vi "Re-tag Larvae v2 (SubVI).vi"(0 "Image Size":T2={"Height"=512, "Width"=512} {"Width" step=8; "Height" step=8}, 1 "BG SUB TH":i16=20, 2 "Subtract BG":bool, 3 "BG Image":u8[][](array[numeric]), 4 "vReset":refnum<queue>, 5 "Data In":T1, 6 "Range":cluster{"Lower value":u8, "Upper value":u8}={"Lower value"=100, "Upper value"=255}, 7 "flipFlag":refnum<queue>, 8 "Box Side":cluster{"Low":u32, "High":u32}={"Low"=16, "High"=96}, 10 "Box W + L":cluster{"Low":u32, "High":u32}={"Low"=40, "High"=150}, 12 "Area":cluster{"Low":u32, "High":u32}={"Low"=448, "High"=1280}) -> (14 "# of Objects":i32, 16 "BBOX Array":u64[](array[numeric]), 19 "HT LOC":u64[](array[numeric]))   [LabVIEW 2020]
uses:
  Controls (HOST)/Image Size.ctl
  Controls (HOST)/Data to Disk Bundle.ctl
  <vilib>/vision/NI_Vision_Development_Module.lvlib
panel:
  in  "Range":cluster{"Lower value":u8, "Upper value":u8}={"Lower value"=100, "Upper value"=255}
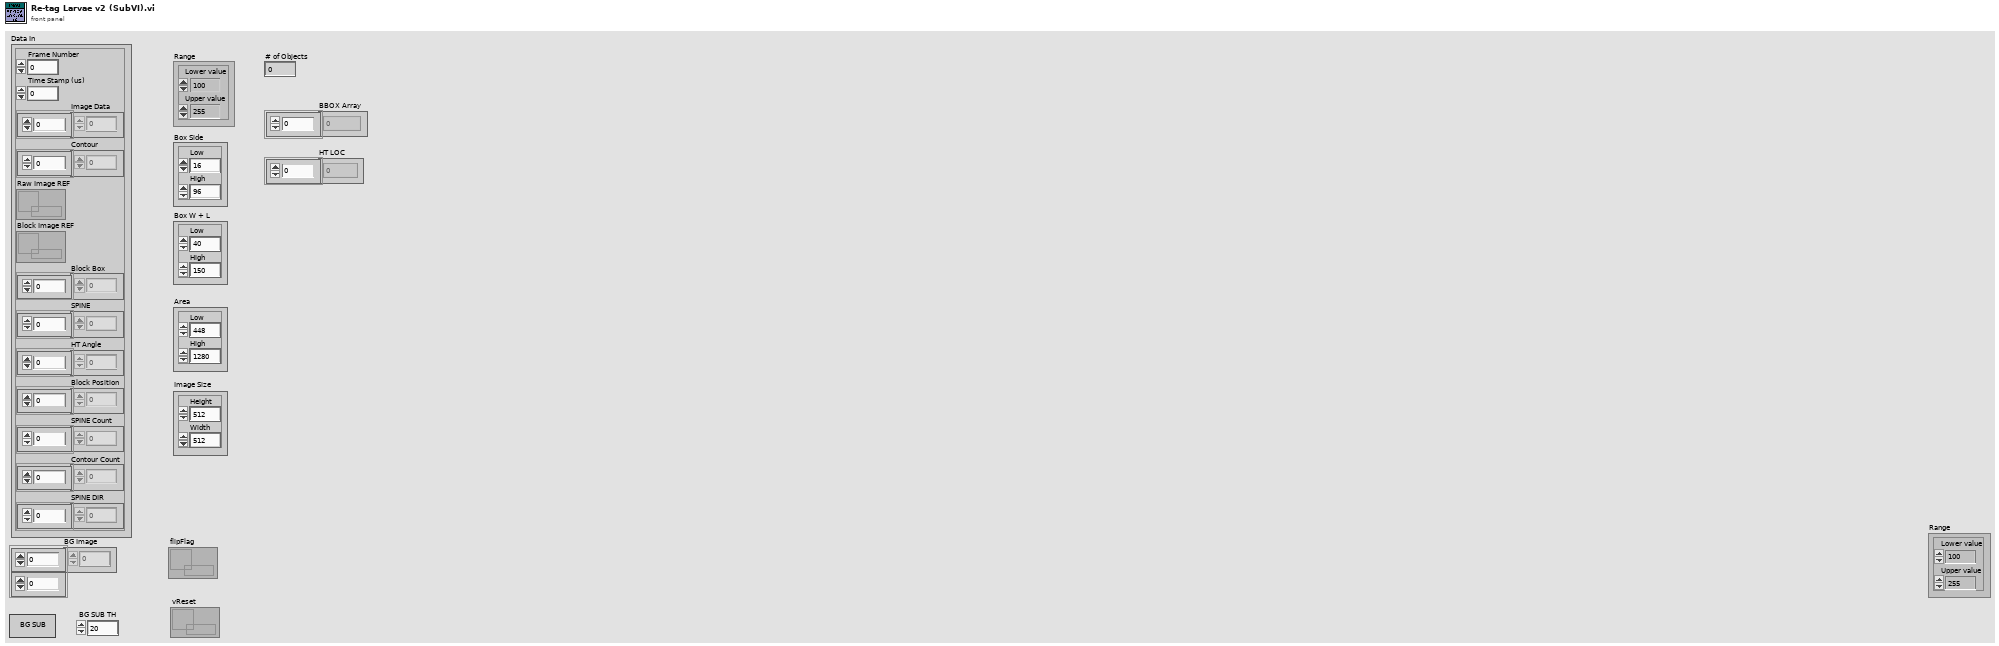
[diagram p1: front panel]
types:
  T1 = typedef "Data to Disk Bundle.ctl" = cluster{"Frame Number":u64, "Time Stamp (us)":u64, "Image Data":u64[], "Contour":u32[], "Raw Image REF":refnum<data-value>, "Block Image REF":refnum<data-value>, "Block Box":u64[], "SPINE":u32[], "HT Angle":u64[], "Block Position":u64[], "SPINE Count":u32[], "Contour Count":u32[], "SPINE DIR":u8[]}
  T2 = typedef "Image Size.ctl" = cluster{"Height":u16, "Width":u16}
  T3 = enum16{"big-endian, network order", "native, host order", "little-endian"}
  T4 = typedef "IMAQ Image.ctl" = refnum<image>
  T5 = cluster{"Area":dbl, "Number of Holes":dbl, "Bounding Rect":cluster{"Left":dbl, "Top":dbl, "Right":dbl, "Bottom":dbl}, "Center of Mass":cluster{"X":dbl, "Y":dbl}, "Orientation":dbl, "Dimensions":cluster{"Width":dbl, "Height":dbl}}[]
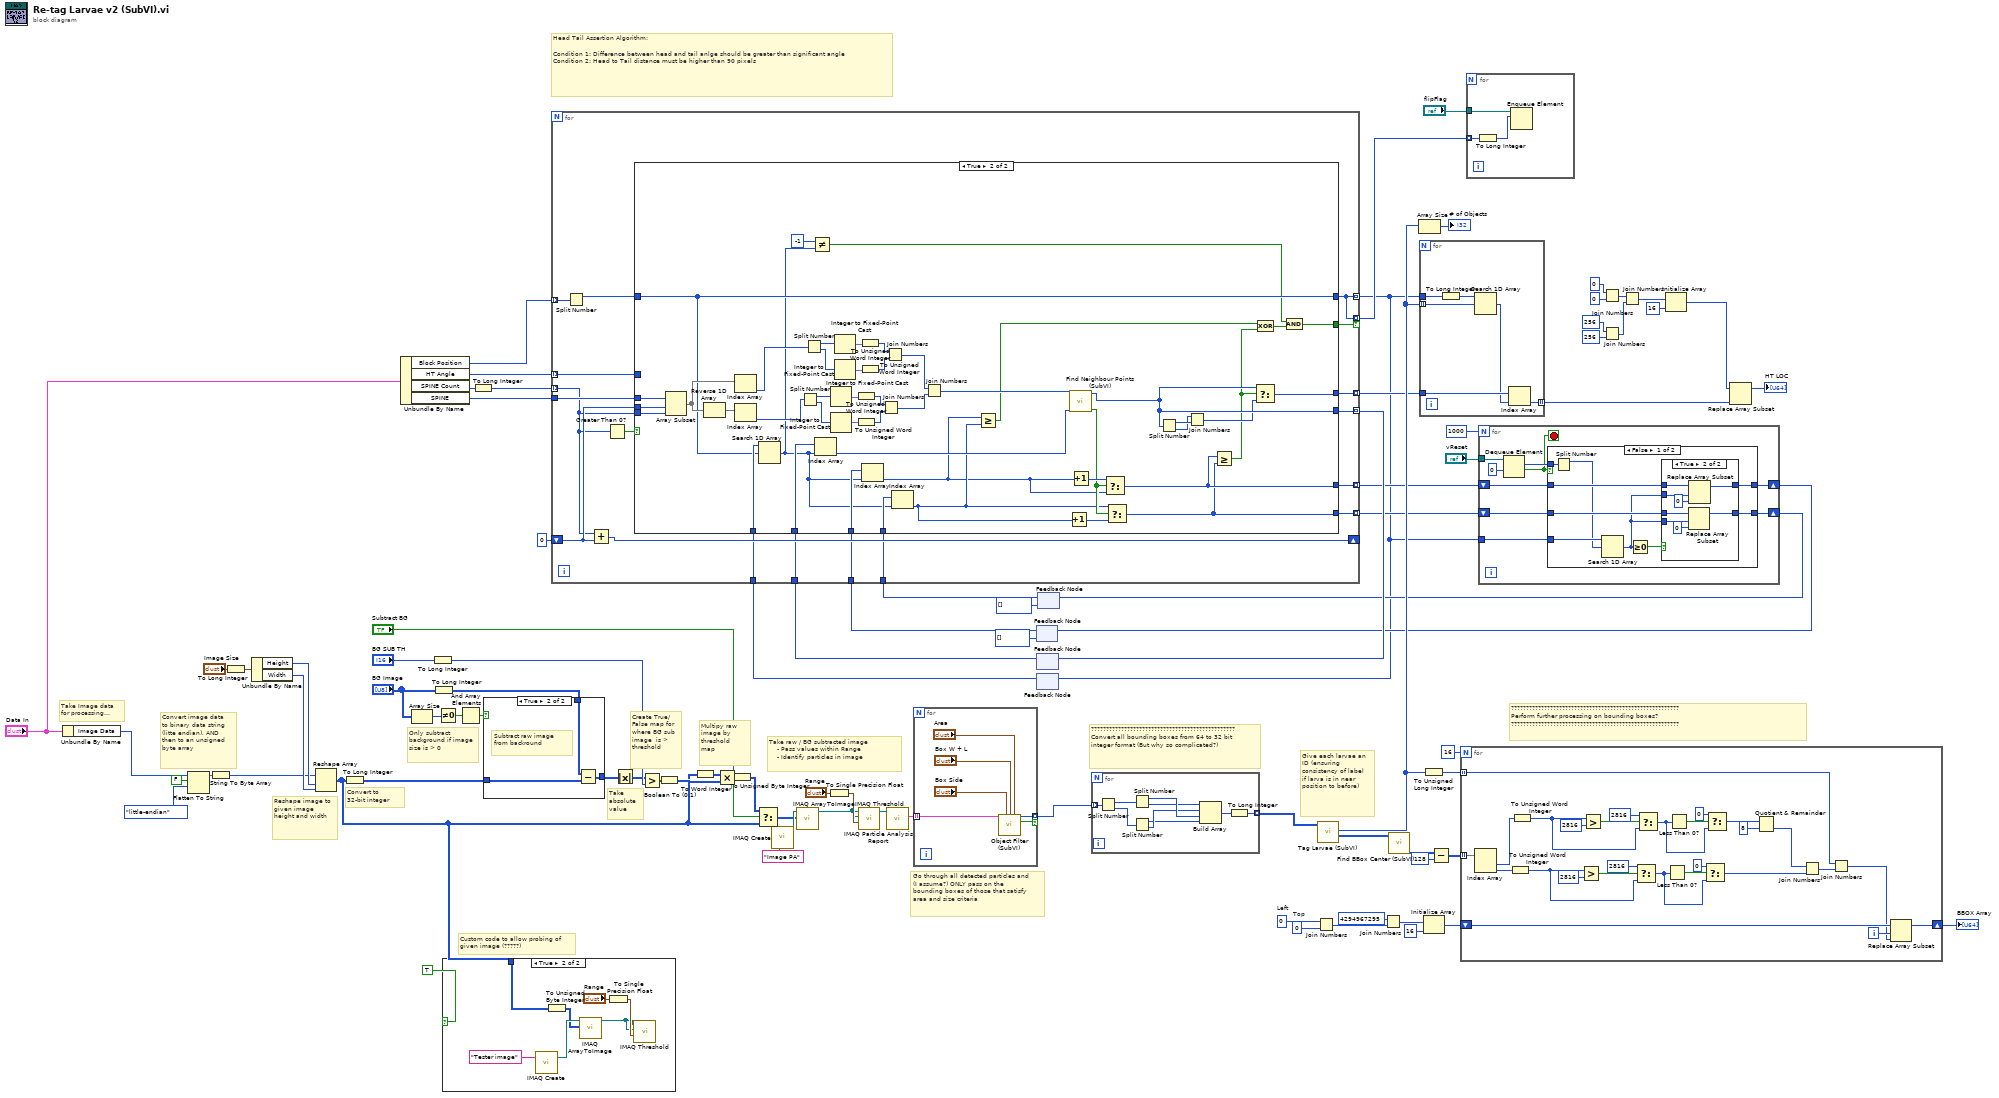
[diagram p0: block diagram]
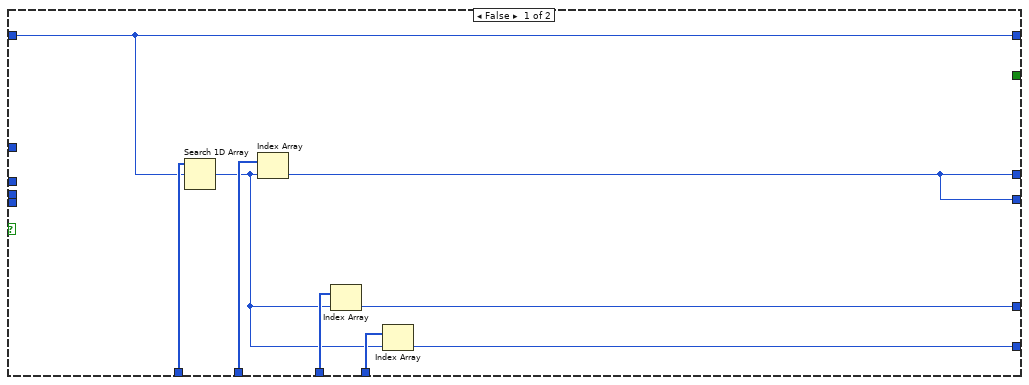
[diagram p5: hidden frame]
diagram:
  w71 = u16 0  # Left
  w67 = u16 0  # Top
  # "????????????????????????????????????????????????????????\nPerform further processing on bounding boxes?\n????????????????????????????????????????????????????????"
  # "Give each larvae an ID (ensuring consistency of label if larva is in near position to before)"
  # "????????????????????????????????????????????????\nConvert all bounding boxes from 64 to 32 bit integer format (But why so complicated?)"
  # "Go through all detected particles and (I assume?) ONLY pass on the bounding boxes of those that satisfy area and size criteria"
  # "Take raw / BG subtracted image\n    - Pass values within Range\n    - Identify particles in image"
  # "Multipy raw image by threshold map"
  # "Create True/False map for where BG sub image  is > threshold"
  # "Take absolute value"
  # "Custom code to allow probing of given image (?????)"
  # "Only subtract background if image size is > 0"
  # "Convert to 32-bit integer"
  # "Reshape image to given image height and width"
  # "Convert image data to binary data string (litte endian), AND then to an unsigned byte array"
  # "Take Image data for processing..."
  # "Head Tail Assertion Algorithm:\n\nCondition 1: Difference between head and tail anlge should be greater than significant angle\nCondition 2: Head to Tail distance must be higher than 90 pixels"
  n1 = Unbundle By Name("Data In") -> ("Image Data"=w58:u64[])
  n2 = Flatten To String(anything=w58, prepend array or string size? (T)=FALSE, byte order (0:big-endian, network order)=T3."little-endian") -> (data string=w55:string)  [unwired: 1 in, 2 out]
  n3 = String To Byte Array(string=w55) -> (unsigned byte array=w45:u8[])
  n4 = To Long Integer(number="Image Size") -> (32bit integer=w51:cluster{"Height":i32, "Width":i32})
  n5 = Unbundle By Name(w51) -> ("Height"=w53:i32, "Width"=w52:i32)
  n6 = Reshape Array(w45, w53, w52) -> (w1:u8[][])
  n7 = To Long Integer(number=w1) -> (32bit integer=w64:i32[][])
  n8 = Unbundle By Name("Data In") -> ("Block Position"=w40:u64[], "HT Angle"=w24:u64[], "SPINE Count"=w44:u32[], "SPINE"=w43:u32[])
  n9 = Array Size(array="BG Image") -> (size(s)=w48:i32[])
  n10 = To Long Integer(number="BG SUB TH") -> (32bit integer=w59:i32)
  n11 = To Long Integer(number="BG Image") -> (32bit integer=w63:i32[][])
  n12 = Not Equal To 0?(x=w48) -> (x != 0?=w47:bool[])
  n13 = case shown="True" TRUE {
    tunnel: w1 -> [_ w93]
    frame False {
    }
    frame True {
      n14 = call "IMAQ Create"("Image Name"="Tester image") -> ("New Image"=w94:T4)  [unwired: 4 in, 1 out]
      n15 = To Unsigned Byte Integer(number=w93) -> (unsigned 8bit integer=w92:u8[][])
      n16 = call "IMAQ ArrayToImage"("Image Pixels (U8)"=w92, "Image"=w94) -> ("Image Out"=w89:T4)  [unwired: 8 in, 1 out]
      n17 = To Single Precision Float(number="Range") -> (single precision float=w90:cluster{"Lower value":sgl, "Upper value":sgl})
      n18 = call "IMAQ Threshold"("Range"=w90, "Image Dst"=w89, "Image Src"=w89) -> ()  [unwired: 7 in, 2 out]
    }
  }
  n19 = And Array Elements(Boolean array=w47) -> (logical AND=w46:bool)
  n20 = To Long Integer(number=w44) -> (32bit integer=w41:i32[])
  n21 = case shown="True" w46 {
    tunnel: w64 -> [w96 w99]
    tunnel: w63 -> [_ w98]
    tunnel: [w96 w97] -> w4
    frame False {
    }
    frame True {
      # "Subtract raw image from backround"
      n22 = Subtract(x=w98, y=w99) -> (x-y=w97:i32[][])
    }
  }
  n23 = Absolute Value(x=w4) -> (abs(x)=w3:i32[][])
  n24 = Greater?(x=w3, y=w59) -> (0:w61:bool[][])
  n25 = Boolean To (0,1)(Boolean=w61) -> (0, 1=w8:i16[][])
  n26 = To Word Integer(number=w1) -> (16bit integer=w7:i16[][])
  n27 = Multiply(x=w7, y=w8) -> (x*y=w6:i16[][])
  n28 = To Unsigned Byte Integer(number=w6) -> (unsigned 8bit integer=w5:u8[][])
  n29 = Select(t=w5, s="Subtract BG", f=w1) -> (s? t:f=w50:u8[][])
  n30 = call "IMAQ Create"("Image Name"="Image PA") -> ("New Image"=w80:T4)  [unwired: 4 in, 1 out]
  n31 = call "IMAQ ArrayToImage"("Image Pixels (U8)"=w50, "Image"=w80) -> ("Image Out"=w82:T4)  [unwired: 8 in, 1 out]
  n32 = To Single Precision Float(number="Range") -> (single precision float=w88:cluster{"Lower value":sgl, "Upper value":sgl})
  n33 = call "IMAQ Threshold"("Range"=w88, "Image Dst"=w82, "Image Src"=w82) -> ("Image Dst Out"=w81:T4)  [unwired: 7 in, 1 out]
  n34 = call "IMAQ Particle Analysis Report"("Image"=w81) -> ("Particle Reports (Pixels)"=w84:T5)  [unwired: 5 in, 5 out]
  n35 = for {
    tunnel: w84 -> [w101] mode=indexing
    tunnel: [w105] -> w85 mode=indexing if=w100
    n36 = call "Object Filter (SubVI).vi"("Particle Report"=w101, "Box Side"="Box Side", "Box W + L"="Box W + L", "Area"="Area") -> ("Bounding Box"=w105:u64, "Data Valid"=w100:bool)  [unwired: 10 in]
  }
  n37 = feedback #1(i32[] []) -> (w23:i32[])
  n38 = feedback #2() -> (w26:u64[])  [unwired: 1 in]
  n39 = feedback #3() -> (w28:u32[])  [unwired: 1 in]
  n40 = feedback #4(i32[] []) -> (w20:i32[])
  n41 = for {
    tunnel: w41 -> [w117] mode=indexing
    tunnel: w43 -> [w122]
    shift-right: [w123] -> _
    shift-left: 0 ("Numeric Control") -> [w121]
    tunnel: [w120] -> w27 mode=indexing
    tunnel: w40 -> [w119] mode=indexing
    tunnel: w28 -> [w116]
    tunnel: w26 -> [w115]
    tunnel: [w107] -> w10 mode=indexing
    tunnel: w24 -> [w108] mode=indexing
    tunnel: [w113] -> w16 mode=indexing
    tunnel: w23 -> [w112]
    tunnel: w20 -> [w111]
    tunnel: [w110] -> w15 mode=indexing
    tunnel: [w109] -> w19 mode=indexing
    tunnel: [w107] -> w14 mode=indexing if=w106
    n42 = Split Number(x=w119) -> (hi(x)=w114:u32)  [unwired: 1 out]
    n43 = Add(x=w117, y=w121) -> (x+y=w123:i32)
    n44 = Greater Than 0?(x=w117) -> (x > 0?=w118:bool)
    n45 = case shown="True" w118 {
      tunnel: w122 -> [_ w179]
      tunnel: w117 -> [_ w178]
      tunnel: w121 -> [_ w177]
      tunnel: [w124 w166] -> w120
      tunnel: w116 -> [w132 w174]
      tunnel: w115 -> [w131 w173]
      tunnel: [w130 w172] -> w107
      tunnel: w114 -> [w130 w172]
      tunnel: [w128 w143] -> w113
      tunnel: w112 -> [w129 w170]
      tunnel: w111 -> [w127 w169]
      tunnel: [w125 w142] -> w110
      tunnel: [w124 w164] -> w109
      tunnel: w108 -> [_ _]
      tunnel: [_ w133] -> w106
      frame False {
        n46 = Search 1D Array(1D array=w132, element=w130) -> (index of element=w126:i32)  [unwired: 1 in]
        n47 = Index Array(array=w131, index=w126) -> (element=w124:u64)
        n48 = Index Array(array=w129, index=w126) -> (element=w128:i32)
        n49 = Index Array(array=w127, index=w126) -> (element=w125:i32)
      }
      frame True {
        n50 = Array Subset(array=w179, index=w177, length=w178) -> (w175:u32[])
        n51 = Reverse 1D Array(array=w175) -> (reversed array=w176:u32[])
        n52 = Index Array(array=w175) -> (element=w156:u32)  [unwired: 1 in]
        n53 = Index Array(array=w176) -> (element=w145:u32)  [unwired: 1 in]
        n54 = Search 1D Array(1D array=w174, element=w172) -> (index of element=w137:i32)  [unwired: 1 in]
        n55 = Split Number(x=w145) -> (hi(x)=w150:u16, lo(x)=w151:u16)
        n56 = Split Number(x=w156) -> (hi(x)=w155:u16, lo(x)=w154:u16)
        n57 = Not Equal?(x=-1, y=w137) -> (x != y?=w134:bool)
        n58 = Index Array(array=w173, index=w137) -> (element=w167:u64)
        n59 = Integer to Fixed-Point Cast(integer=w150) -> (fixed-point=w148:fxp<+,16,9>)  [unwired: 1 in]
        n60 = Integer to Fixed-Point Cast(integer=w151) -> (fixed-point=w149:fxp<+,16,9>)  [unwired: 1 in]
        n61 = Integer to Fixed-Point Cast(integer=w155) -> (fixed-point=w158:fxp<+,16,9>)  [unwired: 1 in]
        n62 = Integer to Fixed-Point Cast(integer=w154) -> (fixed-point=w157:fxp<+,16,9>)  [unwired: 1 in]
        n63 = To Unsigned Word Integer(number=w148) -> (unsigned 16bit integer=w146:u16)
        n64 = To Unsigned Word Integer(number=w149) -> (unsigned 16bit integer=w147:u16)
        n65 = To Unsigned Word Integer(number=w158) -> (unsigned 16bit integer=w160:u16)
        n66 = To Unsigned Word Integer(number=w157) -> (unsigned 16bit integer=w159:u16)
        n67 = Index Array(array=w170, index=w137) -> (element=w140:i32)
        n68 = Join Numbers(hi=w146, lo=w147) -> ((hi.lo)=w144:u32)
        n69 = Join Numbers(hi=w160, lo=w159) -> ((hi.lo)=w153:u32)
        n70 = Index Array(array=w169, index=w137) -> (element=w141:i32)
        n71 = Join Numbers(hi=w153, lo=w144) -> ((hi.lo)=w152:u64)
        n72 = Greater Or Equal?(x=w140, y=w141) -> (x >= y?=w138:bool)
        n73 = Increment(x=w141) -> (x+1=w168:i32)
        n74 = call "Find Neighbour Points (SubVI).vi"("Previous HT Position"=w167, "Current HT Position"=w152) -> ("Increment Vote"=w165:bool, "Neighbor Point"=w164:u64)  [unwired: 8 in]
        n75 = Increment(x=w140) -> (x+1=w171:i32)
        n76 = Select(t=w171, s=w165, f=w140) -> (s? t:f=w143:i32)
        n77 = Select(t=w141, s=w165, f=w168) -> (s? t:f=w142:i32)
        n78 = Split Number(x=w164) -> (hi(x)=w163:u32, lo(x)=w162:u32)
        n79 = Join Numbers(hi=w162, lo=w163) -> ((hi.lo)=w161:u64)
        n80 = Greater Or Equal?(x=w143, y=w142) -> (x >= y?=w139:bool)
        n81 = Exclusive Or(1:w139, 2:w138) -> (0:w135:bool)
        n82 = Select(t=w164, s=w139, f=w161) -> (s? t:f=w166:u64)
        n83 = And(x=w134, y=w135) -> (x .and. y?=w133:bool)
      }
    }
  }
  n84 = feedback-in #2(w19) -> ()
  n85 = feedback-in #3(w10) -> ()
  n86 = for {
    tunnel: w85 -> [w188] mode=indexing
    tunnel: [w180] -> w65 mode=indexing
    n87 = Split Number(x=w188) -> (hi(x)=w187:u32, lo(x)=w186:u32)
    n88 = Split Number(x=w187) -> (hi(x)=w185:u16, lo(x)=w184:u16)
    n89 = Split Number(x=w186) -> (hi(x)=w182:u16, lo(x)=w183:u16)
    n90 = Build Array(w184, w183, w185, w182) -> (w181:u16[])
    n91 = To Long Integer(number=w181) -> (32bit integer=w180:i32[])
  }
  n92 = Join Numbers(hi=w71, lo=w67) -> ((hi.lo)=w68:u32)
  n93 = call "Tag Larvae (SubVI).vi"("Array in"=w65) -> ("Bounding Box"=w74:i32[][], "Current ID"=w39:i32[])  [unwired: 8 in, 1 out]
  n94 = Join Numbers(hi=u32 4294967295, lo=w68) -> ((hi.lo)=w69:u64)
  n95 = call "Find BBox Center (SubVI).vi"("BBox Array In"=w74) -> ("Center Array"=w75:i32[][])  [unwired: 9 in, 1 out]
  n96 = Array Size(array=w39) -> (size(s)=→"# of Objects":i32)
  n97 = for {
    tunnel: w39 -> [w193] mode=indexing
    tunnel: w10 -> [w194]
    tunnel: w27 -> [w191]
    tunnel: [w190] -> w30 mode=indexing
    n98 = To Long Integer(number=w194) -> (32bit integer=w192:i32[])
    n99 = Search 1D Array(1D array=w192, element=w193) -> (index of element=w189:i32)  [unwired: 1 in]
    n100 = Index Array(array=w191, index=w189) -> (element=w190:u64)
  }
  n101 = To Unsigned Long Integer(number=w39) -> (unsigned 32bit integer=w87:u32[])
  n102 = Initialize Array(w69, 16 ("dimension size")) -> (w72:u64[])
  n103 = Subtract(x=w75, y=128) -> (x-y=w76:i32[][])
  n104 = for {
    N: 16 -> [_]
    shift-right: [w220] -> w78
    shift-left: w72 -> [w221]
    tunnel: w76 -> [w218] mode=indexing
    tunnel: w87 -> [w196] mode=indexing
    i -> [w219]
    n105 = Index Array(array=w218) -> (element #1=w200:i32, element #2=w201:i32)  [unwired: 2 in]
    n106 = To Unsigned Word Integer(number=w201) -> (unsigned 16bit integer=w211:u16)
    n107 = To Unsigned Word Integer(number=w200) -> (unsigned 16bit integer=w210:u16)
    n108 = Greater?(x=w211, y=u16 2816) -> (0:w217:bool)
    n109 = Greater?(x=w210, y=u16 2816) -> (0:w204:bool)
    n110 = Select(t=u16 2816 ("y"), s=w217, f=w211) -> (s? t:f=w213:u16)
    n111 = Select(t=u16 2816 ("y"), s=w204, f=w210) -> (s? t:f=w208:u16)
    n112 = Less Than 0?(x=w213) -> (x < 0?=w214:bool)
    n113 = Less Than 0?(x=w208) -> (x < 0?=w207:bool)
    n114 = Select(t=u16 0 ("y"), s=w214, f=w213) -> (s? t:f=w198:u16)
    n115 = Select(t=u16 0 ("y"), s=w207, f=w208) -> (s? t:f=w203:u16)
    n116 = Quotient & Remainder(x=w203, y=u16 8) -> (floor(x/y)=w199:u16)  [unwired: 1 out]
    n117 = Join Numbers(hi=w199, lo=w198) -> ((hi.lo)=w197:u32)
    n118 = Join Numbers(hi=w196, lo=w197) -> ((hi.lo)=w195:u64)
    n119 = Replace Array Subset(array=w221, new element=w195, index=w219) -> (w220:u64[])
  }
  "BBOX Array" <- w78
  n120 = for {
    tunnel: w14 -> [w223] mode=indexing
    tunnel: "flipFlag" -> [w224]
    n121 = To Long Integer(number=w223) -> (32bit integer=w222:i32)
    n122 = Enqueue Element(queue=w224, element=w222) -> ()  [unwired: 2 in, 3 out]
  }
  n123 = for {
    N: 1000 -> [_]
    tunnel: "vReset" -> [w233]
    shift-right: [w228] -> w11
    shift-left: w15 -> [w229]
    shift-right: [w227] -> w12
    shift-left: w16 -> [w230]
    tunnel: w10 -> [w231]
    stop <- w225 stop-if-true
    n124 = Dequeue Element(queue=w233, timeout in ms (-1)=0) -> (element=w226:u64, timed out?=w225:bool)  [unwired: 1 in, 2 out]
    n125 = case shown="False" w225 {
      tunnel: w226 -> [w241 _]
      tunnel: w231 -> [w242 _]
      tunnel: w230 -> [w240 w253]
      tunnel: w229 -> [w237 w254]
      tunnel: [w236 w254] -> w228
      tunnel: [w238 w253] -> w227
      frame False {
        n126 = Split Number(x=w241) -> (hi(x)=w234:u32)  [unwired: 1 out]
        n127 = Search 1D Array(1D array=w242, element=w234) -> (index of element=w235:i32)  [unwired: 1 in]
        n128 = Greater Or Equal To 0?(x=w235) -> (x >= 0?=w239:bool)
        n129 = case shown="True" w239 {
          tunnel: w240 -> [w244 w252]
          tunnel: [w244 w251] -> w238
          tunnel: w237 -> [w243 w249]
          tunnel: [w243 w248] -> w236
          tunnel: w235 -> [_ w250]
          tunnel: w235 -> [_ w247]
          frame False {
          }
          frame True {
            n130 = Replace Array Subset(array=w249, new element=0 ("new element/subarray"), index=w247) -> (w248:i32[])
            n131 = Replace Array Subset(array=w252, new element=0 ("new element/subarray"), index=w250) -> (w251:i32[])
          }
        }
      }
      frame True {
      }
    }
  }
  n132 = feedback-in #1(w12) -> ()
  n133 = feedback-in #4(w11) -> ()
  n134 = Join Numbers(hi=u16 0 ("Numeric Control"), lo=u16 0 ("Numeric Control")) -> ((hi.lo)=w34:u32)
  n135 = Join Numbers(hi=u16 256 ("Numeric Control"), lo=u16 256 ("Numeric Control")) -> ((hi.lo)=w33:u32)
  n136 = Join Numbers(hi=w34, lo=w33) -> ((hi.lo)=w32:u64)
  n137 = Initialize Array(w32, 16 ("dimension size")) -> (w25:u64[])
  n138 = Replace Array Subset(array=w25, new element=w30) -> (→"HT LOC":u64[])  [unwired: 1 in]
